vi "joystick_axis_conditioner.vi"(1 "joystick axis":dbl(slide)=1.0 min=-1.0 max=1.0 step=0.01 scale=-1.0..1.0, 2 "Sensitivity":dbl=1.0 format="%#_13g", 3 "Deadband":dbl=0.15) -> (0 "output":dbl)   [LabVIEW 2017]
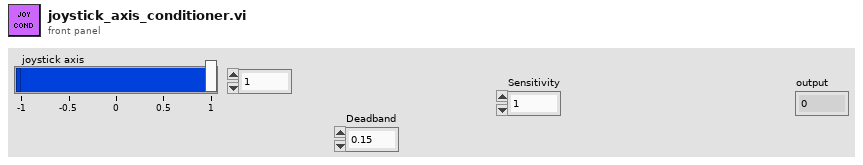
[diagram p1: front panel]
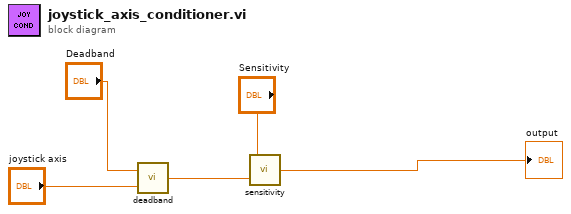
[diagram p0: block diagram]
diagram:
  n1 = call "deadband.vi"("joystick axis"="joystick axis", "Deadband"="Deadband") -> ("deadbanded_output"=w3:dbl)
  n2 = call "sensitivity.vi"("input"=w3, "Sensitivity"="Sensitivity") -> ("output"=→"output":dbl)
